vi "Class - ResultCntr.SubSectionStart.vi"(8 "error in (no error)":errorcluster, 11 "Class - ResultCntr in":refnum<class "Class - ResultCntr.lvclass">) -> (0 "error out":errorcluster, 1 "ID":string, 3 "Class - ResultCntr out":refnum<class "Class - ResultCntr.lvclass">)   [LabVIEW 2024, in "EQMF.lvlib" / "Results.lvlib" / "Class - ResultCntr.lvclass"]
uses:
  Class - ResultCntr.lvclass
  Class - ResultCntr.lvclass/Class - ResultCntr.ctl
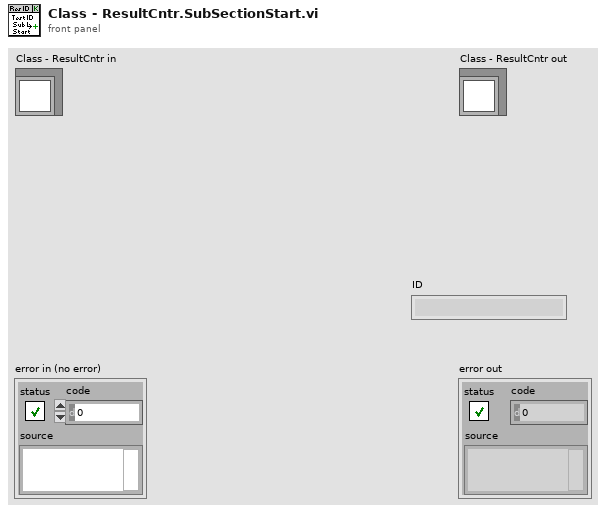
[diagram p1: front panel]
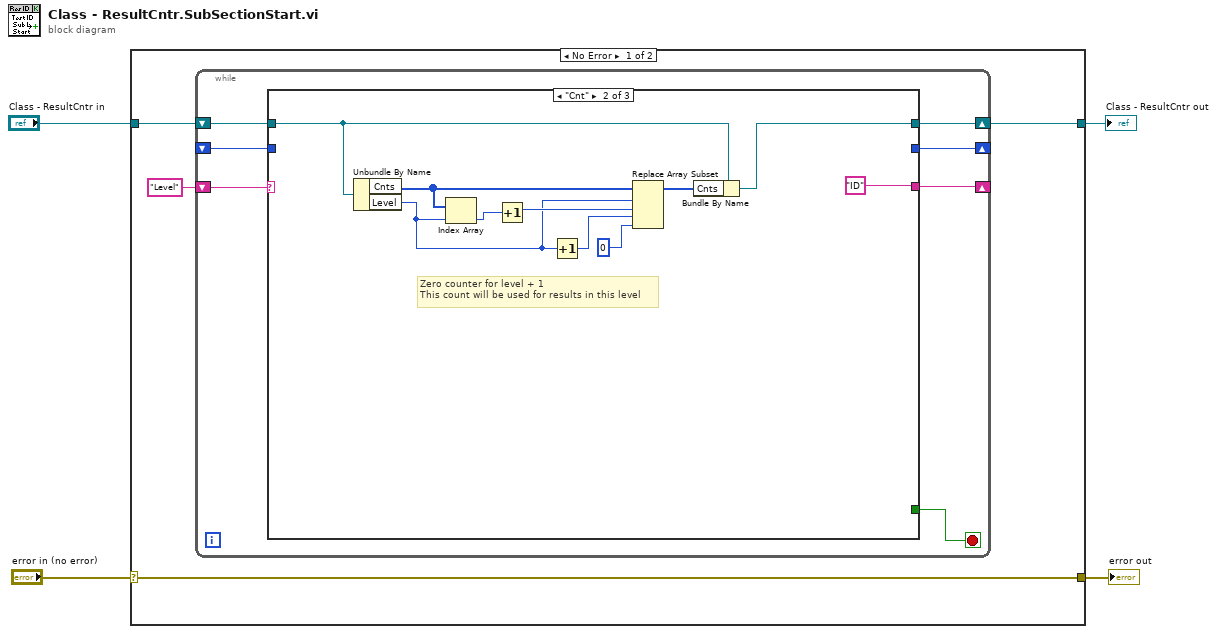
[diagram p0: block diagram]
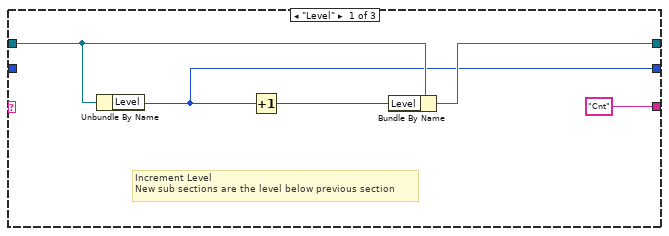
[diagram p2: hidden frame]
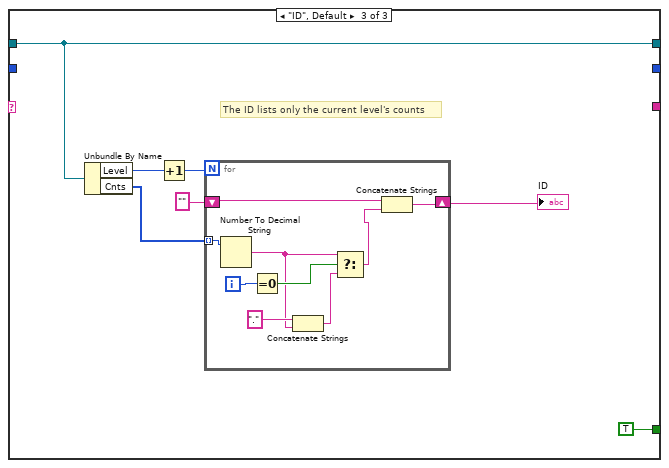
[diagram p3: hidden frame]
diagram:
  n1 = case shown="No Error" "error in (no error)" {
    selector: "error in (no error)" -> [w8 w48]
    tunnel: [w8 w48] -> w3
    tunnel: [w5 w47] -> w1
    tunnel: "Class - ResultCntr in" -> [w7 w47]
    frame No Error {
      n2 = while {
        shift-right: [w13] -> w5
        shift-left: w7 -> [w14]
        shift-right: [w12] -> _
        shift-left: "Level" -> [w15]
        shift-right: [w10] -> _
        shift-left: _ -> [w9]
        stop <- w11 stop-if-true
        n3 = case shown="\"Cnt\"" w15 {
          tunnel: w14 -> [w19 w28 w34]
          tunnel: [w18 w27 w34] -> w13
          tunnel: ["Cnt" "ID" _] -> w12
          tunnel: [_ _ TRUE] -> w11
          tunnel: [w16 _ _] -> w10
          tunnel: w9 -> [_ _ _]
          frame "Level" {
            # "Increment Level\nNew sub sections are the level below previous section"
            n4 = Unbundle By Name(w19) -> ("Level"=w16:i32)
            n5 = Increment(x=w16) -> (x+1=w17:i32)
            n6 = Bundle By Name(cluster=w19, "Level"=w17) -> (w18:refnum<class "Class - ResultCntr.lvclass">)
          }
          frame "Cnt" {
            # "Zero counter for level + 1\nThis count will be used for results in this level"
            n7 = Unbundle By Name(w28) -> ("Cnts"=w22:i32[], "Level"=w21:i32)
            n8 = Index Array(array=w22, index=w21) -> (element=w23:i32)
            n9 = Increment(x=w23) -> (x+1=w24:i32)
            n10 = Increment(x=w21) -> (x+1=w25:i32)
            n11 = Replace Array Subset(array=w22, new element #1=w24, index #1=w21, new element #2=0 ("new element/subarray"), index #2=w25) -> (w29:i32[])
            n12 = Bundle By Name(cluster=w28, "Cnts"=w29) -> (w27:refnum<class "Class - ResultCntr.lvclass">)
          }
          frame "ID", Default {
            # "The ID lists only the current level's counts"
            n13 = Unbundle By Name(w34) -> ("Level"=w33:i32, "Cnts"=w32:i32[])
            n14 = Increment(x=w33) -> (x+1=w36:i32)
            n15 = for {
              N: w36 -> [_]
              tunnel: w32 -> [w45] mode=indexing
              shift-right: [w40] -> w31
              shift-left: "" -> [w39]
              i -> [w46]
              n16 = Number To Decimal String(number=w45) -> (decimal integer string=w41:string)  [unwired: 1 in]
              n17 = Equal To 0?(x=w46) -> (x = 0?=w42:bool)
              n18 = Concatenate Strings(".", w41) -> (w43:string)
              n19 = Select(t=w41, s=w42, f=w43) -> (s? t:f=w38:string)
              n20 = Concatenate Strings(w39, w38) -> (w40:string)
            }
            "ID" <- w31
          }
        }
      }
    }
    frame Error {
    }
  }
  "error out" <- w3
  "Class - ResultCntr out" <- w1
